vi "Facade.vi"(0 "Data In":T4, 2 "Display State In":T2, 3 "Container State":T3) -> (6 "Data Out":T4, 7 "Display State Out":T2, 8 "Action":T1)   [LabVIEW 2020, in "Noise.xctl"]
uses:
  Noise.xctl
  Data.vi
  Classes/Waveforms/Noise/Noise.lvclass
  <vilib>/_xctls/Container State.ctl
  State.vi
  <vilib>/_xctls/Action.ctl
  Classes/Waveforms/Noise/Noise.lvclass/Noise.ctl
  Classes/Waveforms/Noise/Read Seed.vi
  Classes/Waveforms/Noise/Read Tokens.vi
  Classes/Waveforms/Noise/Read InvFilt.vi
  Classes/Waveforms/Noise/Read Aweight.vi
  Classes/Waveforms/Noise/Write Seed.vi
  Classes/Waveforms/Noise/Write Tokens.vi
  Classes/Waveforms/Noise/Write InvFilt.vi
  Classes/Waveforms/Noise/Write Aweight.vi
  <vilib>/_xctls/XControlSupport.lvlib
panel:
  in  "Weights":u16(ring) items=["White", "Pink"]
  in  "Inverse filter":bool caption="Acoustic system compensation"
  in  "A-weight":bool caption="Audiogram compensation"
  in  "Seed":i32
  in  "Tokens":i32 min=0 step=1
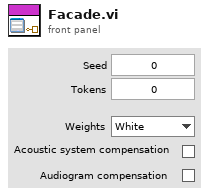
[diagram p1: front panel]
types:
  T1 = typedef "XControlSupport.lvlib/Action.ctl" = cluster{"Data Changed?":bool, "State Changed?":bool, "Action Name":string}
  T2 = typedef "Noise.xctl/State.vi" = cluster{"Numeric":dbl}
  T3 = typedef "XControlSupport.lvlib/Container State.ctl" = cluster{"Indicator?":bool, "Run Mode?":bool, " Refnum":refnum<vi>}
  T4 = typedef "Noise.xctl/Data.vi" = refnum<class "Noise.lvclass">
  T5 = typedef "Noise.lvclass/Weighting.ctl" = enum16{"White", "Pink"}
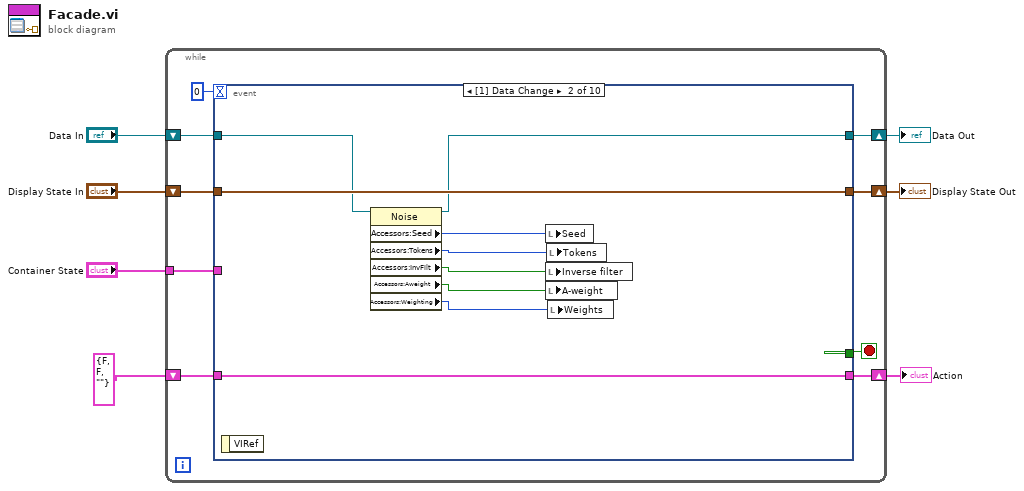
[diagram p0: block diagram]
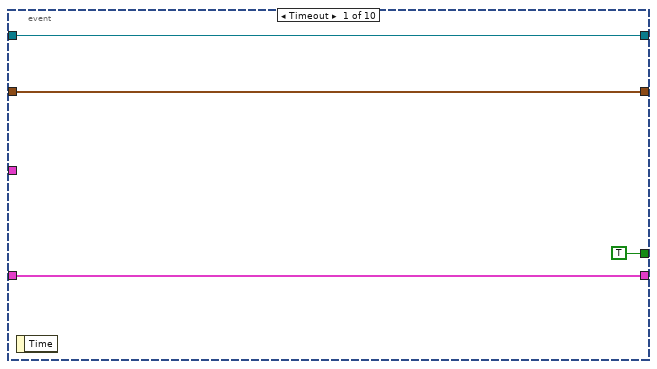
[diagram p2: hidden frame]
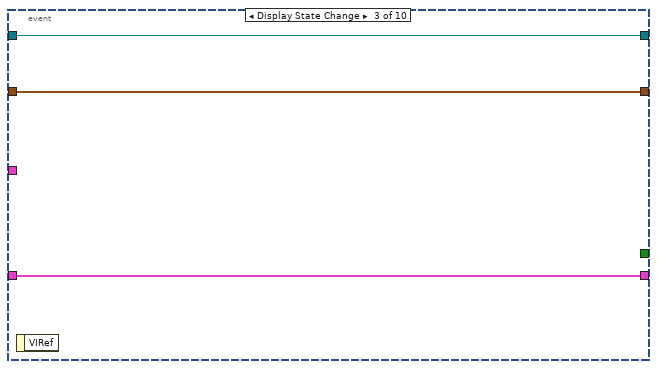
[diagram p3: hidden frame]
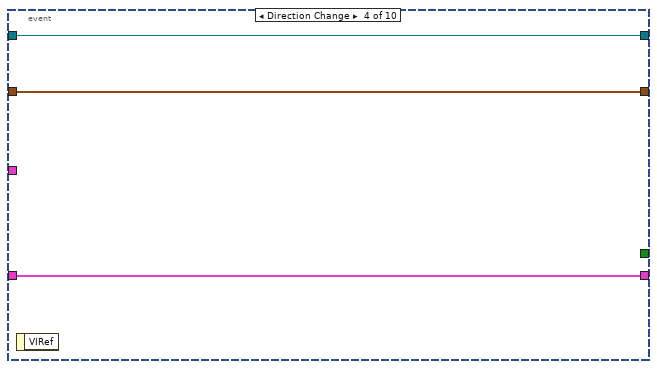
[diagram p4: hidden frame]
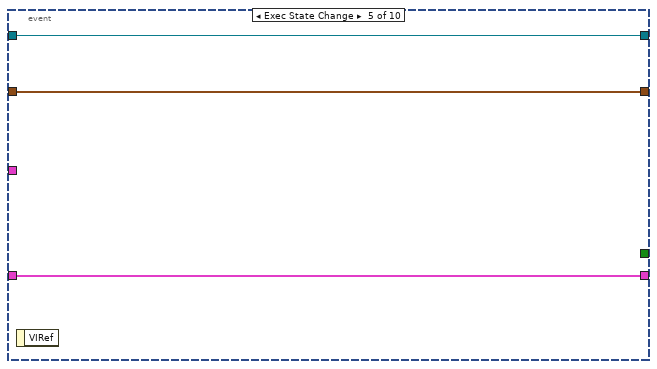
[diagram p5: hidden frame]
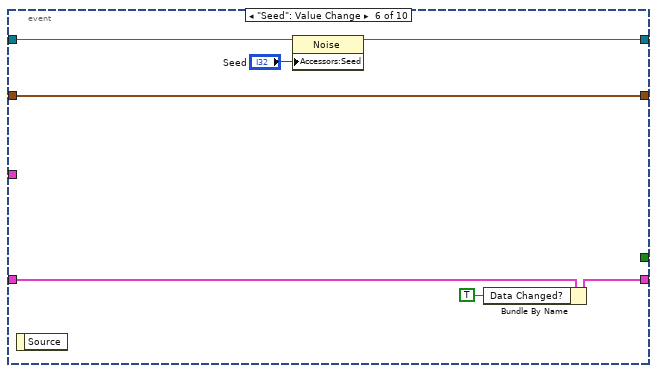
[diagram p6: hidden frame]
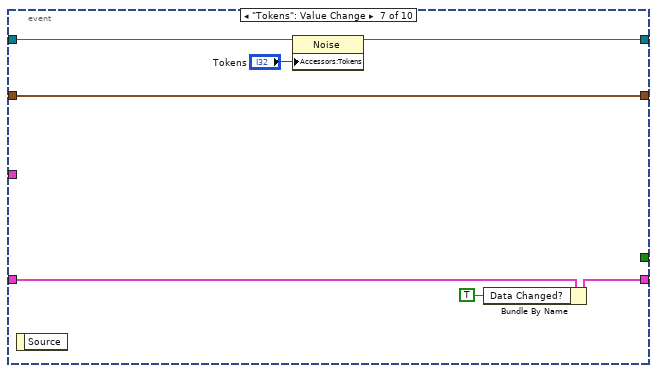
[diagram p7: hidden frame]
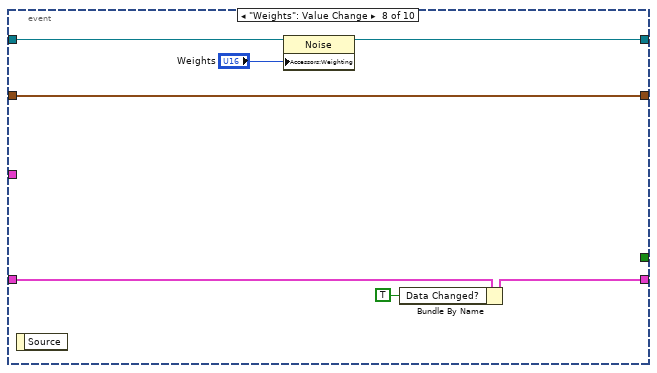
[diagram p8: hidden frame]
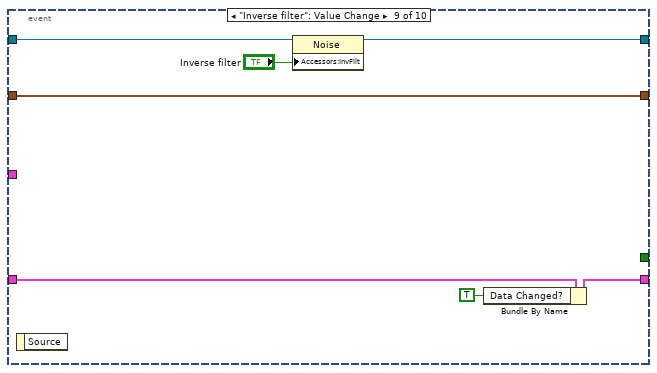
[diagram p9: hidden frame]
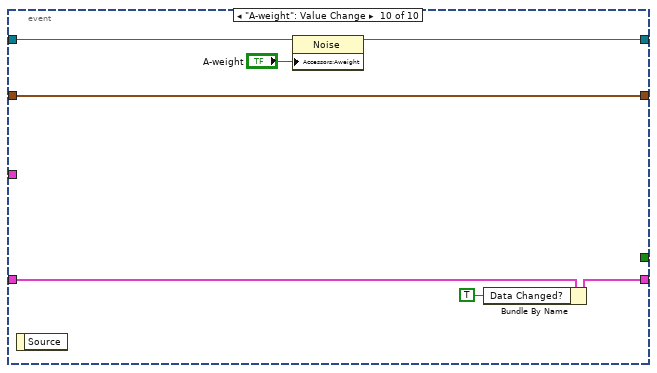
[diagram p10: hidden frame]
diagram:
  n1 = while {
    shift-right: [w15] -> w4
    shift-left: "Display State In" -> [w16]
    tunnel: "Container State" -> [w12]
    shift-right: [w10] -> w7
    shift-left: "Data In" -> [w11]
    shift-right: [w8] -> w2
    shift-left: T1 {"Data Changed?"=FALSE, "State Changed?"=FALSE, "Action Name"=""} ("Action") -> [w9]
    stop <- w14 stop-if-true
    n2 = event shown="[1] Data Change" {
      selector: _ -> [_ _ _ _ _ _ _ _ _ _]
      dyn-events: _ -> [_ _ _ _ _ _ _ _ _ _]
      timeout: 0 -> [_ _ _ _ _ _ _ _ _ _]
      tunnel: w16 -> [w18 w29 w32 w35 w38 w45 w52 w59 w66 w73]
      tunnel: [w18 w29 w32 w35 w38 w45 w52 w59 w66 w73] -> w15
      tunnel: [TRUE _ _ _ _ _ _ _ _ _] -> w14
      tunnel: w12 -> [_ _ _ _ _ _ _ _ _ _]
      tunnel: w11 -> [w17 w27 w31 w34 w37 w44 w51 w58 w65 w72]
      tunnel: [w17 w22 w31 w34 w37 w40 w47 w56 w61 w68] -> w10
      tunnel: [w19 w28 w30 w33 w36 w42 w49 w55 w63 w70] -> w8
      tunnel: w9 -> [w19 w28 w30 w33 w36 w43 w50 w57 w64 w71]
      event Timeout {
        n3 = event-data() -> ()  [unwired: 1 in, 1 out]
      }
      event Data Change {
        n4 = event-data() -> ()  [unwired: 1 in, 1 out]
        n5 = property class="Noise"(reference=w27) -> (reference out=w22:T4, "Accessors:Seed"=w26:i32, "Accessors:Tokens"=w25:i32, "Accessors:InvFilt"=w24:bool, "Accessors:Aweight"=w23:bool, "Accessors:Weighting"=w21:T5)  [unwired: 1 in, 1 out]
        n6 = local write "Seed"(w26) -> ()
        n7 = local write "Inverse filter"(w24) -> ()
        n8 = local write "A-weight"(w23) -> ()
        n9 = local write "Tokens"(w25) -> ()
        n10 = local write "Weights"(w21) -> ()
      }
      event Display State Change {
        n11 = event-data() -> ()  [unwired: 1 in, 1 out]
      }
      event Direction Change {
        n12 = event-data() -> ()  [unwired: 1 in, 1 out]
      }
      event Exec State Change {
        n13 = event-data() -> ()  [unwired: 1 in, 1 out]
      }
      event "Seed": Value Change {
        n14 = event-data() -> ()  [unwired: 1 in, 1 out]
        n15 = property class="Noise"(reference=w44, "Accessors:Seed"="Seed") -> (reference out=w40:T4)  [unwired: 1 in, 1 out]
        n16 = Bundle By Name(cluster=w43, "Data Changed?"=TRUE) -> (w42:T1)
      }
      event "Tokens": Value Change {
        n17 = event-data() -> ()  [unwired: 1 in, 1 out]
        n18 = property class="Noise"(reference=w51, "Accessors:Tokens"="Tokens") -> (reference out=w47:T4)  [unwired: 1 in, 1 out]
        n19 = Bundle By Name(cluster=w50, "Data Changed?"=TRUE) -> (w49:T1)
      }
      event "Weights": Value Change {
        n20 = event-data() -> ()  [unwired: 1 in, 1 out]
        n21 = property class="Noise"(reference=w58, "Accessors:Weighting"="Weights") -> (reference out=w56:T4)  [unwired: 1 in, 1 out]
        n22 = Bundle By Name(cluster=w57, "Data Changed?"=TRUE) -> (w55:T1)
      }
      event "Inverse filter": Value Change {
        n23 = event-data() -> ()  [unwired: 1 in, 1 out]
        n24 = property class="Noise"(reference=w65, "Accessors:InvFilt"="Inverse filter") -> (reference out=w61:T4)  [unwired: 1 in, 1 out]
        n25 = Bundle By Name(cluster=w64, "Data Changed?"=TRUE) -> (w63:T1)
      }
      event "A-weight": Value Change {
        n26 = event-data() -> ()  [unwired: 1 in, 1 out]
        n27 = property class="Noise"(reference=w72, "Accessors:Aweight"="A-weight") -> (reference out=w68:T4)  [unwired: 1 in, 1 out]
        n28 = Bundle By Name(cluster=w71, "Data Changed?"=TRUE) -> (w70:T1)
      }
    }
  }
  "Display State Out" <- w4
  "Data Out" <- w7
  "Action" <- w2
